vi "Actor Core.vi"(8 "error in (no error)":errorcluster, 11 "Operator UI.lvclass":refnum<class "Controller UI.lvclass">) -> (0 "error out":errorcluster, 3 "Actor Framework.lvlib:Actor":refnum<class "Actor.lvclass">)   [LabVIEW 2016, in "Controller UI.lvlib" / "Controller UI.lvclass"]
doc: "This is Actor Core.vi, the main message handling loop for Actors. An actor usually just sits in this loop and processes messages as they arrive. Any error returned by the message Do.vi call will stop the loop, with error code 43 as the cannonical signal to stop with no error sent to caller. Descendants may override that in Handle Error.vi."
uses:
  <userlib>/Common Components/Controller UI/Controller UI.lvclass
  <vilib>/ActorFramework/Stop Msg/Stop Msg.lvclass
  <userlib>/Common Components/Controller UI/Messages/Send Run Function Message/Send Run Function Message.lvclass
  <userlib>/Common Components/Controller UI/Messages/Send Get Hardware Info Message/Send Get Hardware Info Message.lvclass
  <userlib>/Common Components/Controller UI/Messages/Prompt User for Path to load/Prompt User for File Path to Load From.lvclass
  <userlib>/Common Components/Controller UI/Messages/Ask Controller to Launch Results UI Msg/Ask Controller to Launch Results UI Msg.lvclass
  <vilib>/ActorFramework/Actor/Actor.lvclass
  <userlib>/Common Components/User Interface/UI.lvclass
  C:/Program Files (x86)/National Instruments/LabVIEW 2016/vi.lib/ActorFramework/Actor/Actor.lvclass
  C:/Program Files (x86)/National Instruments/LabVIEW 2016/user.lib/Common Components/User Interface/UI.lvclass
panel:
  in  "Master/Slave":enum32{"Master", "Slave"}(radio)
  in  "about":bool
  in  "Load New Function":bool
  in  "Show FP?":bool
  in  "Stop Button":bool
  in  "Run":bool
  in  "Functions":u16(ring)
  in  "Tab Control":enum32{"Status", "Results"}(tab)
  in  "Status Display":string
  in  "View Results":bool
  in  "Results Listbox":i32(listbox)
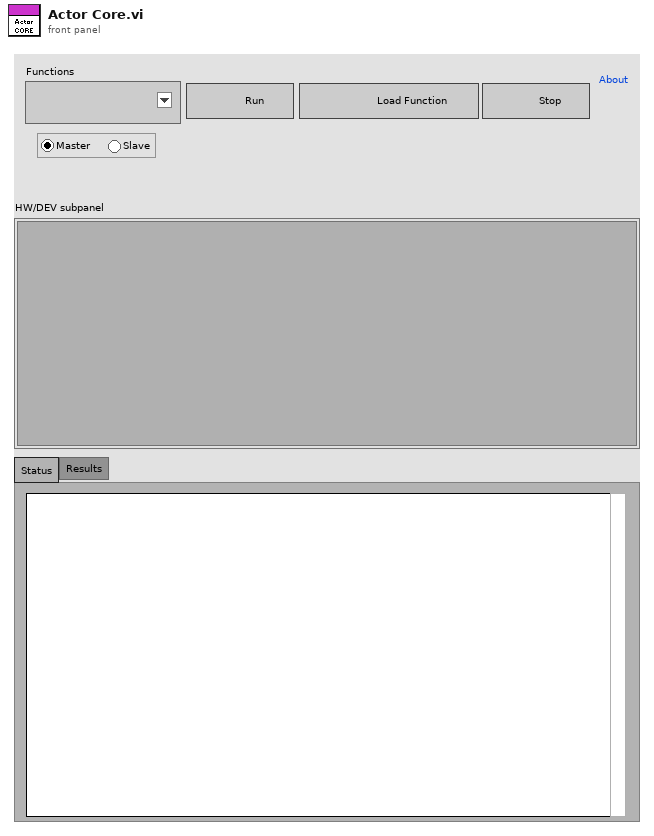
[diagram p1: front panel]
types:
  T1 = enum8{"Enabled", "Disabled", "Disabled and Grayed Out"}
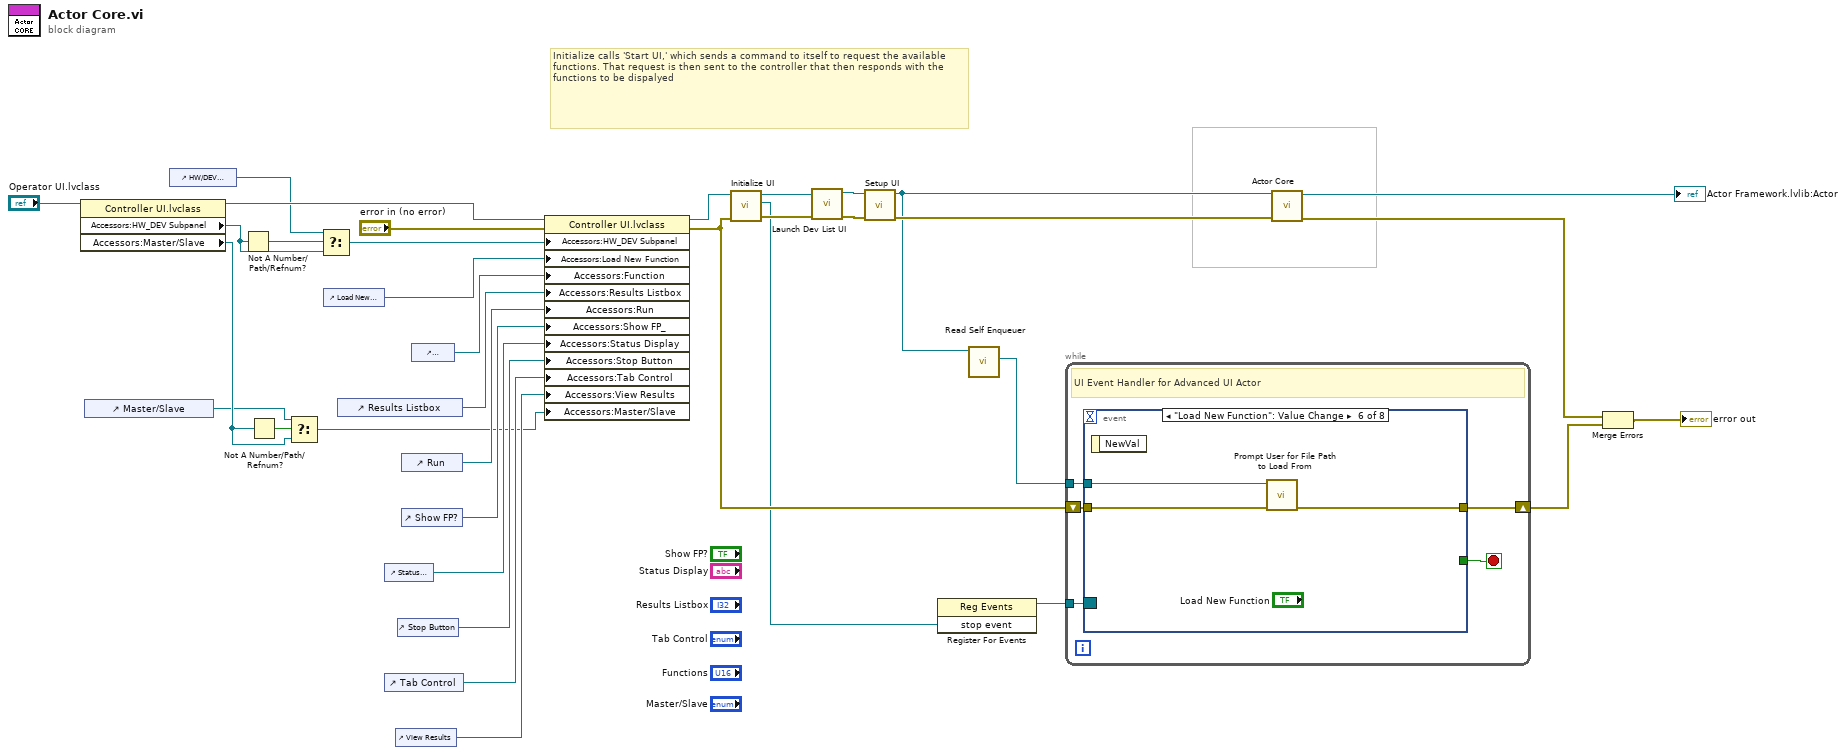
[diagram p0: block diagram]
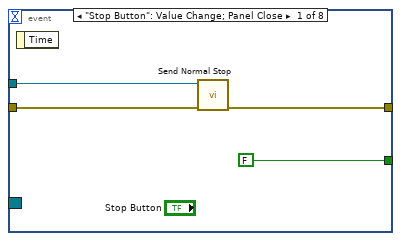
[diagram p2: hidden frame]
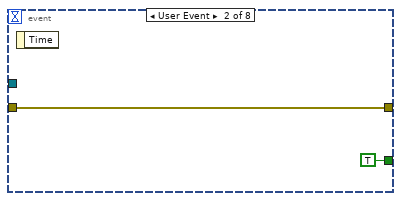
[diagram p3: hidden frame]
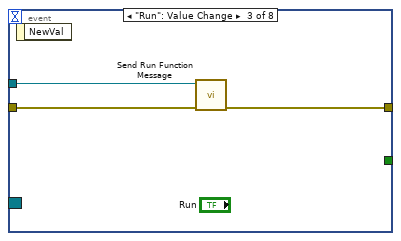
[diagram p4: hidden frame]
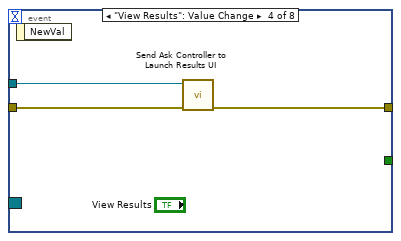
[diagram p5: hidden frame]
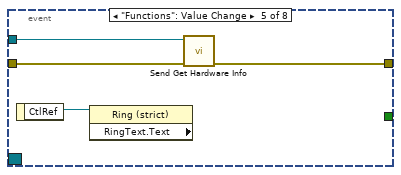
[diagram p6: hidden frame]
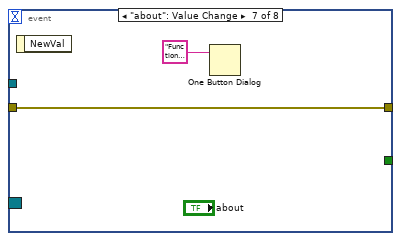
[diagram p7: hidden frame]
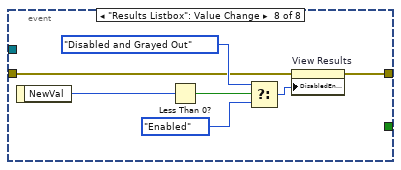
[diagram p8: hidden frame]
diagram:
  # "Initialize calls 'Start UI,' which sends a command to itself to request the available functions. That request is then sent to the controller that then responds with the functions to be dispalyed"
  n1 = property class="Controller UI.lvclass"(reference="Operator UI.lvclass") -> (reference out=w14:refnum<class "Controller UI.lvclass">, "Accessors:HW_DEV Subpanel"=w11:refnum<vi>, "Accessors:Master/Slave"=w3:refnum<vi>)  [unwired: 1 in, 1 out]
  n2 = control-ref of="Master/Slave"() -> (w2:refnum<vi>)
  n3 = control-ref of="HW/DEV subpanel"() -> (w12:refnum<vi>)
  n4 = Not A Number/Path/Refnum?(number/path/refnum=w11) -> (NaN/Path/Refnum?=w13:bool)
  n5 = Not A Number/Path/Refnum?(number/path/refnum=w3) -> (NaN/Path/Refnum?=w4:bool)
  n6 = Select(t=w2, s=w4, f=w3) -> (s? t:f=w1:refnum<vi>)
  n7 = Select(t=w12, s=w13, f=w11) -> (s? t:f=w10:refnum<vi>)
  n8 = control-ref of="Load New Function"() -> (w22:refnum<vi>)
  n9 = control-ref of="Results Listbox"() -> (w23:refnum<vi>)
  n10 = control-ref of="Status Display"() -> (w27:refnum<vi>)
  n11 = control-ref of="Tab Control"() -> (w25:refnum<vi>)
  n12 = control-ref of="View Results"() -> (w24:refnum<vi>)
  n13 = control-ref of="Stop Button"() -> (w26:refnum<vi>)
  n14 = control-ref of="Run"() -> (w20:refnum<vi>)
  n15 = control-ref of="Show FP?"() -> (w28:refnum<vi>)
  n16 = control-ref of="Functions"() -> (w21:refnum<vi>)
  n17 = property class="Controller UI.lvclass"(reference=w14, error in="error in (no error)", "Accessors:HW_DEV Subpanel"=w10, "Accessors:Load New Function"=w22, "Accessors:Function"=w21, "Accessors:Results Listbox"=w23, "Accessors:Run"=w20, "Accessors:Show FP_"=w28, "Accessors:Status Display"=w27, "Accessors:Stop Button"=w26, "Accessors:Tab Control"=w25, "Accessors:View Results"=w24, "Accessors:Master/Slave"=w1) -> (reference out=w18:refnum<class "Controller UI.lvclass">, error out=w16:errorcluster)
  n18 = call <userlib>:"Initialize UI.vi"("error in (no error)"=w16, "UI in"=w18) -> ("error out"=w17:errorcluster, "stop event"=w8:refnum<user-event>, "UI out"=w6:refnum<class "Controller UI.lvclass">)  [unwired: 7 in]
  n19 = call <userlib>:"Launch Dev List UI.vi"("error in (no error)"=w17, "Controller UI in"=w6) -> ("error out"=w7:errorcluster, "Controller UI out"=w5:refnum<class "Controller UI.lvclass">)  [unwired: 8 in]
  n20 = call-dynamic "Setup UI.vi"("error in (no error)"=w7, "Operator UI in"=w5) -> ("error out"=w15:errorcluster, "Operator UI out"=w9:refnum<class "Controller UI.lvclass">)  [unwired: 8 in]
  n21 = register-events(w8) -> (reference out=w30:refnum<event-registration>)  [unwired: 2 in, 1 out]
  n22 = call <vilib>:"Read Self Enqueuer.vi"("Actor"=w9) -> ("Self Enqueuer"=w34:refnum<class "Message Enqueuer.lvclass">)  [unwired: 10 in]
  n23 = while {
    tunnel: w34 -> [w39]
    tunnel: w30 -> [w38]
    shift-right: [w36] -> w33
    shift-left: w16 -> [w37]
    stop <- w40 stop-if-true
    # "UI Event Handler for Advanced UI Actor"
    n24 = event shown="[5] \"Load New Function\": Value Change" {
      selector: w38 -> [_ _ _ _ _ _ _ _]
      dyn-events: _ -> [_ _ _ _ _ _ _ _]
      timeout: _ -> [_ _ _ _ _ _ _ _]
      tunnel: [FALSE TRUE _ _ _ _ _ _] -> w40
      tunnel: w39 -> [w43 _ w49 w52 w56 w59 _ _]
      tunnel: w37 -> [w42 w45 w48 w51 w55 w58 w60 w63]
      tunnel: [w41 w45 w47 w50 w54 w57 w60 w62] -> w36
      event "Stop Button": Value Change; Panel Close {
        n25 = event-data() -> ()  [unwired: 1 in, 1 out]
        n26 = call <vilib>:"Send Normal Stop.vi"("error in (no error)"=w42, "Message Enqueuer"=w43) -> ("error out"=w41:errorcluster)  [unwired: 9 in]
      }
      event User Event {
        n27 = event-data() -> ()  [unwired: 1 in, 1 out]
      }
      event "Run": Value Change {
        n28 = event-data() -> ()  [unwired: 1 in, 1 out]
        n29 = call <userlib>:"Send Run Function Message.vi"("error in (no error)"=w48, "Message Enqueuer in"=w49) -> ("error out"=w47:errorcluster)  [unwired: 8 in, 1 out]
      }
      event "View Results": Value Change {
        n30 = event-data() -> ()  [unwired: 1 in, 1 out]
        n31 = call <userlib>:"Send Ask Controller to Launch Results UI.vi"("error in (no error)"=w51, "Message Enqueuer in"=w52) -> ("error out"=w50:errorcluster)  [unwired: 8 in, 1 out]
      }
      event "Functions": Value Change {
        n32 = event-data() -> ("CtlRef"=w53:refnum<vi>)  [unwired: 1 in]
        n33 = property class="Ring (strict)" props=["RingText", "Text"](reference=w53) -> ()  [unwired: 1 in, 3 out]
        n34 = call <userlib>:"Send Get Hardware Info.vi"("error in (no error)"=w55, "Message Enqueuer in"=w56) -> ("error out"=w54:errorcluster)  [unwired: 8 in, 1 out]
      }
      event "Load New Function": Value Change {
        n35 = event-data() -> ()  [unwired: 1 in, 1 out]
        n36 = call <userlib>:"Prompt User for File Path to Load From.vi"("error in (no error)"=w58, "Message Enqueuer in"=w59) -> ("error out"=w57:errorcluster)  [unwired: 8 in, 1 out]
      }
      event "about": Value Change {
        n37 = event-data() -> ()  [unwired: 1 in, 1 out]
        n38 = One Button Dialog(message="Function Manager v2.0\n\nNational Instruments (C) 2013\nWritten in NI LabVIEW 2012 by Elijah Kerry \nElijah.Kerry@ni.com\n\nni.com/largeapps\nekerry.wordpress.com") -> ()  [unwired: 1 in, 1 out]
      }
      event "Results Listbox": Value Change {
        n39 = event-data() -> ("NewVal"=w64:i32)  [unwired: 1 in]
        n40 = Less Than 0?(x=w64) -> (x < 0?=w65:bool)
        n41 = Select(t=T1."Disabled and Grayed Out" ("Disabled"), s=w65, f=T1."Enabled" ("Disabled")) -> (s? t:f=w68:T1)
        n42 = property on="View Results" class="Bool"(error in=w63, "DisabledEnum"=w68) -> (error out=w62:errorcluster)  [unwired: 1 in, 1 out]
      }
    }
  }
  n43 = call-parent "Actor Core.vi"("error in"=w15, "User Interface"=w9) -> ("error out"=w32:errorcluster, "Actor out"=→"Actor Framework.lvlib:Actor":refnum<class "Actor.lvclass">)  [unwired: 8 in]
  n44 = Merge Errors(w32, w33) -> (→"error out":errorcluster)
